vi "setupWaveformFactory.vi"(8 "error in (no error)":errorcluster, 10 "Model in":refnum<class "Model.lvclass">, 11 "Bootloader in":refnum<class "Bootloader.lvclass">) -> (0 "error out":errorcluster, 2 "Model out":refnum<class "Model.lvclass">, 3 "Bootloader out":refnum<class "Bootloader.lvclass">)   [LabVIEW 2015, in "Bootloader.lvclass"]
uses:
  Bootloader.lvclass
  Model/Model.lvclass
  WaveformFactory/WaveformFactory/WaveformFactory.lvclass
  Model/Model.lvclass/Model.ctl
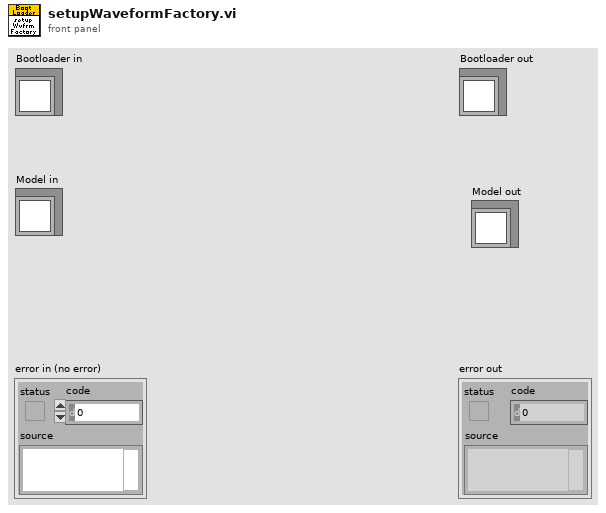
[diagram p1: front panel]
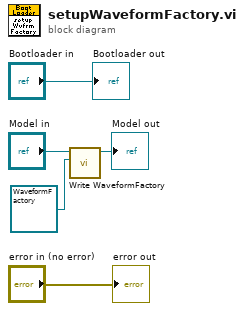
[diagram p0: block diagram]
diagram:
  n1 = call "Write WaveformFactory.vi"("WaveformFactory"=refnum<class "WaveformFactory.lvclass"> refnum ("WaveformFactory.lvclass"), "Model in"="Model in") -> ("Model out"=→"Model out":refnum<class "Model.lvclass">)  [unwired: 9 in]
  "error out" <- "error in (no error)"
  "Bootloader out" <- "Bootloader in"
